vi "Create Subscriber.vi"(8 "error in (no error)":errorcluster, 11 "System Actor in":refnum<class "System Actor.lvclass">) -> (0 "error out":errorcluster, 3 "System Actor out":refnum<class "System Actor.lvclass">)   [LabVIEW 2024, in "System Actor.lvclass"]
uses:
  System Actor.lvclass
  System Actor.lvclass/System Actor.ctl
  Messenger/Mail Strategy/Mail Strategy.lvclass
  Actor Assistant/Observer/Observer.lvclass
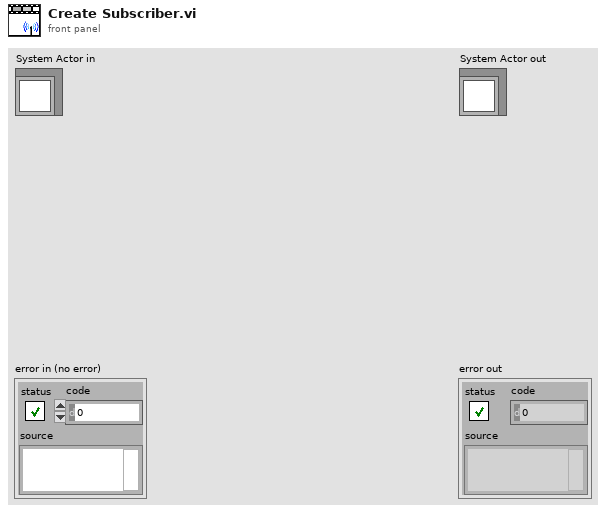
[diagram p1: front panel]
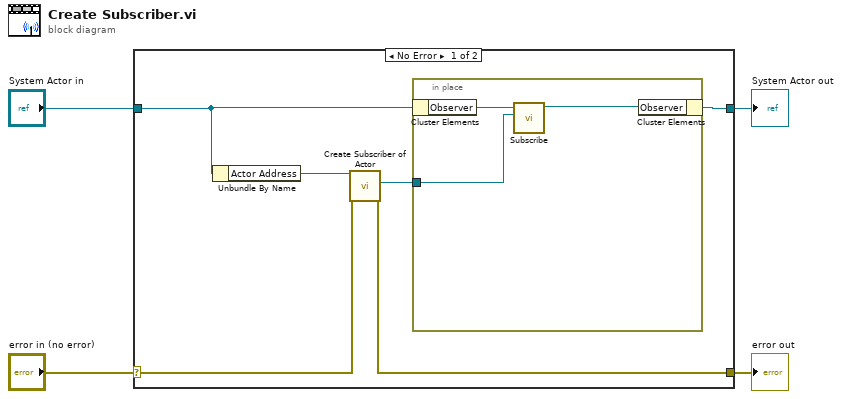
[diagram p0: block diagram]
diagram:
  n1 = case shown="No Error" "error in (no error)" {
    selector: "error in (no error)" -> [w9 w15]
    tunnel: [w8 w15] -> w3
    tunnel: [w6 w14] -> w1
    tunnel: "System Actor in" -> [w7 w14]
    frame No Error {
      n2 = Unbundle By Name(w7) -> ("Actor Address"=w10:refnum<class "Mail Strategy.lvclass">)
      n3 = call-dynamic "Create Subscriber of Actor.vi"("error in (no error)"=w9, "Mail Strategy in"=w10) -> ("error out"=w8:errorcluster, "Subscriber Out"=w5:refnum<class "Subscriber.lvclass">)  [unwired: 7 in, 1 out]
      n4 = in-place {
        in-place-border: w5 -> [w12]
        n5 = in-place-cluster #1(w7) -> ("Observer"=w13:refnum<class "Observer.lvclass">)
        n6 = call-dynamic "Subscribe.vi"("Subscriber In"=w12, "Observer in"=w13) -> ("Observer out"=w11:refnum<class "Observer.lvclass">)  [unwired: 8 in, 1 out]
        n7 = in-place-cluster #1("Observer"=w11) -> (w6:refnum<class "System Actor.lvclass">)
      }
    }
    frame Error {
    }
  }
  "error out" <- w3
  "System Actor out" <- w1
